vi "SelectTrace.vi"(0 "VISA IN":refnum<visa-resource-name>, 5 "error in":errorcluster) -> (14 "VISA Out":refnum<visa-resource-name>, 19 "error out":errorcluster)   [LabVIEW 2018, in "PNA-X.lvlib"]
uses:
  PNA-X.lvlib
panel:
  in  "Trace":i32=1
  in  "Window":i32=1
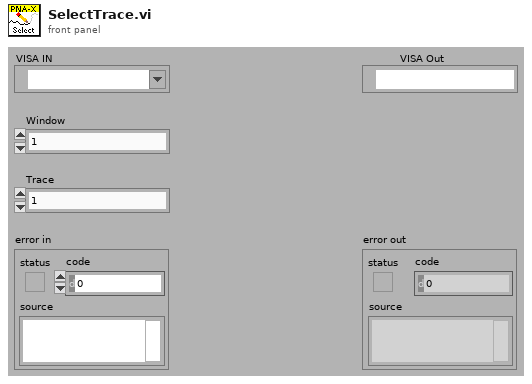
[diagram p1: front panel]
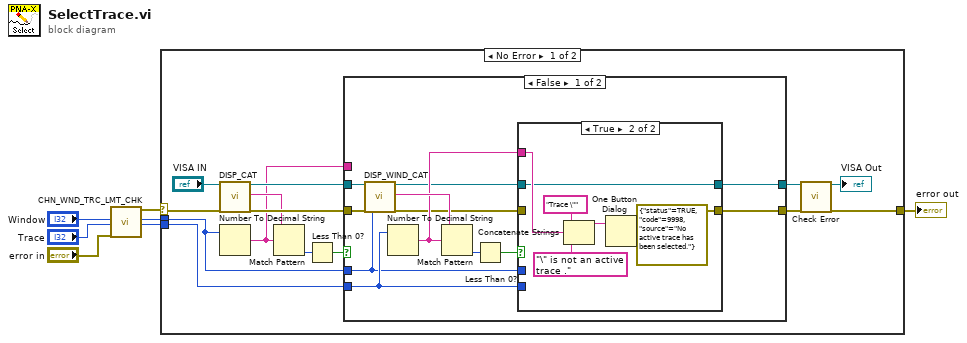
[diagram p0: block diagram]
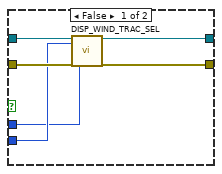
[diagram p2: hidden frame]
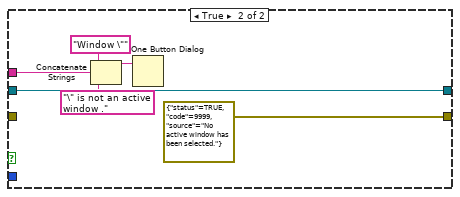
[diagram p3: hidden frame]
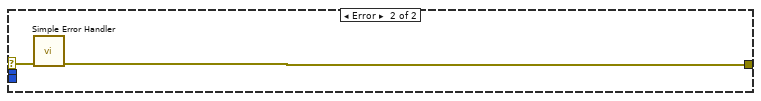
[diagram p4: hidden frame]
diagram:
  n1 = call "CHN_WND_TRC_LMT_CHK.vi"("Window"="Window", "Trace"="Trace", "error in"="error in") -> ("error out"=w3:errorcluster, "Window"=w2:i32, "Trace"=w1:i32)  [unwired: 12 in, 2 out]
  n2 = case shown="No Error" w3 {
    selector: w3 -> [w17 w53]
    tunnel: [w21 w52] -> w5
    tunnel: w2 -> [w8 _]
    tunnel: w1 -> [w9 _]
    frame No Error {
      n3 = call "DISP_CAT.vi"("VISA IN"="VISA IN", "error in"=w17) -> ("VISA Out"=w16:refnum<visa-resource-name>, "Data"=w13:string, "error out"=w18:errorcluster)  [unwired: 15 in]
      n4 = Number To Decimal String(number=w8) -> (decimal integer string=w10:string)  [unwired: 1 in]
      n5 = Match Pattern(string=w13, regular expression=w10) -> (offset past match=w12:i32)  [unwired: 1 in, 3 out]
      n6 = Less Than 0?(x=w12) -> (x < 0?=w11:bool)
      n7 = case shown="False" w11 {
        tunnel: [w26 errorcluster {"status"=TRUE, "code"=9999, "source"="No active window has been selected."} ("error out")] -> w19
        tunnel: w18 -> [w33 _]
        tunnel: w16 -> [w32 w51]
        tunnel: [w24 w51] -> w15
        tunnel: w10 -> [_ w50]
        tunnel: w9 -> [w23 _]
        tunnel: w8 -> [w22 _]
        frame False {
          n8 = call "DISP_WIND_CAT.vi"("VISA IN"=w32, "error in"=w33, "Window"=w22) -> ("VISA Out"=w25:refnum<visa-resource-name>, "Data"=w30:string, "error out"=w27:errorcluster)  [unwired: 14 in]
          n9 = Number To Decimal String(number=w23) -> (decimal integer string=w28:string)  [unwired: 1 in]
          n10 = Match Pattern(string=w30, regular expression=w28) -> (offset past match=w31:i32)  [unwired: 1 in, 3 out]
          n11 = Less Than 0?(x=w31) -> (x < 0?=w29:bool)
          n12 = case shown="True" w29 {
            tunnel: w28 -> [_ w42]
            tunnel: w27 -> [w39 _]
            tunnel: [w38 errorcluster {"status"=TRUE, "code"=9998, "source"="No active trace has been selected."} ("error out")] -> w26
            tunnel: w25 -> [w37 w40]
            tunnel: [w36 w40] -> w24
            tunnel: w23 -> [w35 _]
            tunnel: w22 -> [w34 _]
            frame False {
              n13 = call "DISP_WIND_TRAC_SEL.vi"("VISA IN"=w37, "Trace"=w35, "error in"=w39, "Window"=w34) -> ("VISA Out"=w36:refnum<visa-resource-name>, "error out"=w38:errorcluster)  [unwired: 14 in]
            }
            frame True {
              n14 = Concatenate Strings("Trace \"", w42, "\" is not an active trace .") -> (w43:string)
              n15 = One Button Dialog(message=w43) -> ()  [unwired: 1 in, 1 out]
            }
          }
        }
        frame True {
          n16 = Concatenate Strings("Window \"", w50, "\" is not an active window .") -> (w47:string)
          n17 = One Button Dialog(message=w47) -> ()  [unwired: 1 in, 1 out]
        }
      }
      n18 = call "Check Error.vi"("VISA Resource Name"=w15, "error in (no error)"=w19) -> ("dup VISA session"=→"VISA Out":refnum<visa-resource-name>, "error out"=w21:errorcluster)  [unwired: 16 in]
    }
    frame Error {
      n19 = call <vilib>:"Simple Error Handler.vi"("error in (no error)"=w53) -> ("error out"=w52:errorcluster)  [unwired: 4 in, 4 out]
    }
  }
  "error out" <- w5
